vi "Core Actor - CLOSE - External Queues_Notifiers.vi"(8 "error in (no error)":errorcluster, 11 "Parent_Class in":refnum<class "Message_Distributor_Class.lvclass">) -> (0 "error out":errorcluster, 3 "Parent_Class out":refnum<class "Message_Distributor_Class.lvclass">)   [LabVIEW 2023, in "Actor_Message_Distributor.lvlib" / "Message_Distributor_Class.lvclass"]
uses:
  Message_Distributor_Class.lvclass
  Message_Distributor_Class.lvclass/Message_Distributor_Class.ctl
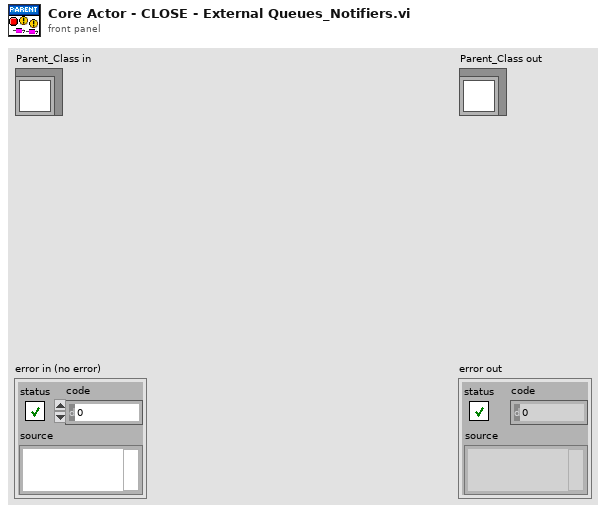
[diagram p1: front panel]
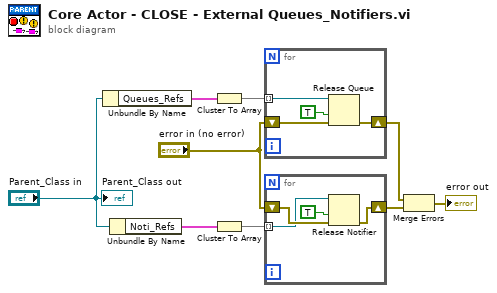
[diagram p0: block diagram]
diagram:
  n1 = Unbundle By Name("Parent_Class in") -> ("Queues_Refs"=w5:cluster{"TX_QUEUE_REF":refnum<queue>})
  n2 = Unbundle By Name("Parent_Class in") -> ("Noti_Refs"=w4:cluster{"TX_NOTI_REF":refnum<notifier>})
  n3 = Cluster To Array(cluster=w5) -> (array=w2:refnum<queue>[])
  n4 = Cluster To Array(cluster=w4) -> (array=w1:refnum<notifier>[])
  n5 = for {
    shift-right: [w11] -> w8
    shift-left: "error in (no error)" -> [w12]
    tunnel: w2 -> [w10] mode=indexing
    n6 = Release Queue(queue=w10, force destroy? (F)=TRUE, error in (no error)=w12) -> (error out=w11:errorcluster)  [unwired: 2 out]
  }
  n7 = for {
    shift-right: [w15] -> w7
    shift-left: "error in (no error)" -> [w16]
    tunnel: w1 -> [w14] mode=indexing
    n8 = Release Notifier(notifier=w14, force destroy? (F)=TRUE, error in (no error)=w16) -> (error out=w15:errorcluster)  [unwired: 2 out]
  }
  n9 = Merge Errors(w8, w7) -> (→"error out":errorcluster)
  "Parent_Class out" <- "Parent_Class in"
